vi "GLdrv_MEAS_OUTP_ORDER.vi"(0 "Connection ID":T1, 11 "error in (no error)":errorcluster) -> (4 "Connection ID Out":T1, 6 "Order out":string, 15 "error out":errorcluster)   [LabVIEW 2017, in "GL860_Driver.lvlib"]
doc: "ACK/ONEコマンドで受信するバイナリデータの並び順を参照します\n例）:MEAS:OUTP:ORDER \"Order = CH1,CH2, .......AlarmOut,Status\"\n詳細はGBDヘッダ仕様書を参照してください"
uses:
  GL860_Driver.lvlib
  ConnectionID.ctl
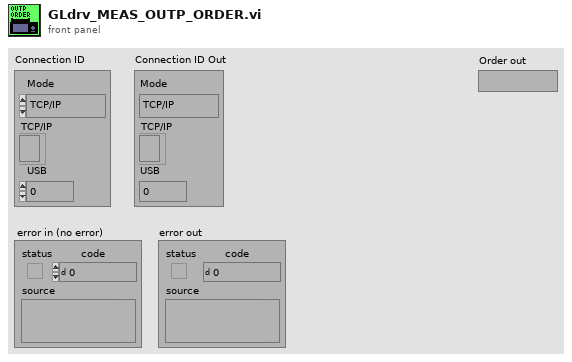
[diagram p1: front panel]
types:
  T1 = typedef "ConnectionID.ctl" = cluster{"Mode":enum16{"TCP/IP", "USB"}, "TCP/IP":refnum<k5>, "USB":i32}
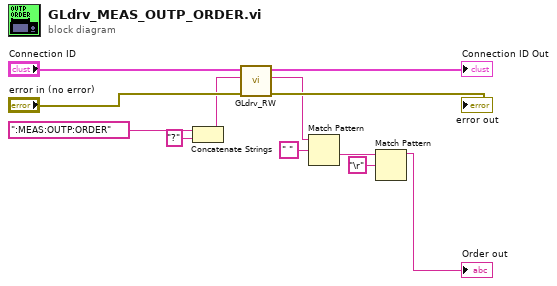
[diagram p0: block diagram]
diagram:
  n1 = Concatenate Strings(":MEAS:OUTP:ORDER" ("Command"), "?" ("string")) -> (w6:string)
  n2 = call "GLdrv_RW.vi"("error in (no error)"="error in (no error)", "data in"=w6, "Connection ID"="Connection ID") -> ("error out"=→"error out":errorcluster, "data out"=w2:string, "Connection ID Out"=→"Connection ID Out":T1)  [unwired: 4 in, 2 out]
  n3 = Match Pattern(string=w2, regular expression=" " ("search string/char (-)")) -> (after substring=w3:string)  [unwired: 4 out]
  n4 = Match Pattern(string=w3, regular expression="\r") -> (before substring=→"Order out":string)  [unwired: 4 out]
